vi "Prepare message set.vi"() -> (1 "Map":T3(c390), 2 "NoMessges":i32[][](array[numeric]), 3 "Array of Tx and Rx messages":T4(array[cluster]) {"ID" format="%.0x"; "DATA[0]" format="%.0x"; "DATA[1]" format="%.0x"; "DATA[2]" format="%.0x"; "DATA[3]" format="%.0x"; "DATA[4]" format="%.0x"; "DATA[5]" format="%.0x"; "DATA[6]" format="%.0x"; "DATA[7]" format="%.0x"})   [LabVIEW 2025]
uses:
  Commands.ctl
  <vilib>/Utility/file.llb/Read Delimited Spreadsheet (string).vi
panel:
  in  "Enum 3":T1=enum."MCU Reset"
  out "key not found?":bool
  out "value":T2 {"Tx und Rx"."DATA[0]" format="%.0x"; "Tx und Rx"."DATA[1]" format="%.0x"; "Tx und Rx"."DATA[2]" format="%.0x"; "Tx und Rx"."DATA[3]" format="%.0x"; "Tx und Rx"."DATA[4]" format="%.0x"; "Tx und Rx"."DATA[5]" format="%.0x"; "Tx und Rx"."DATA[6]" format="%.0x"; "Tx und Rx"."DATA[7]" format="%.0x"}
  in  "stop":bool
  out "Array":bool[](array[boolean])
  out "for debug":string[][](array[string])
  out "all rows":string[][](array[string])
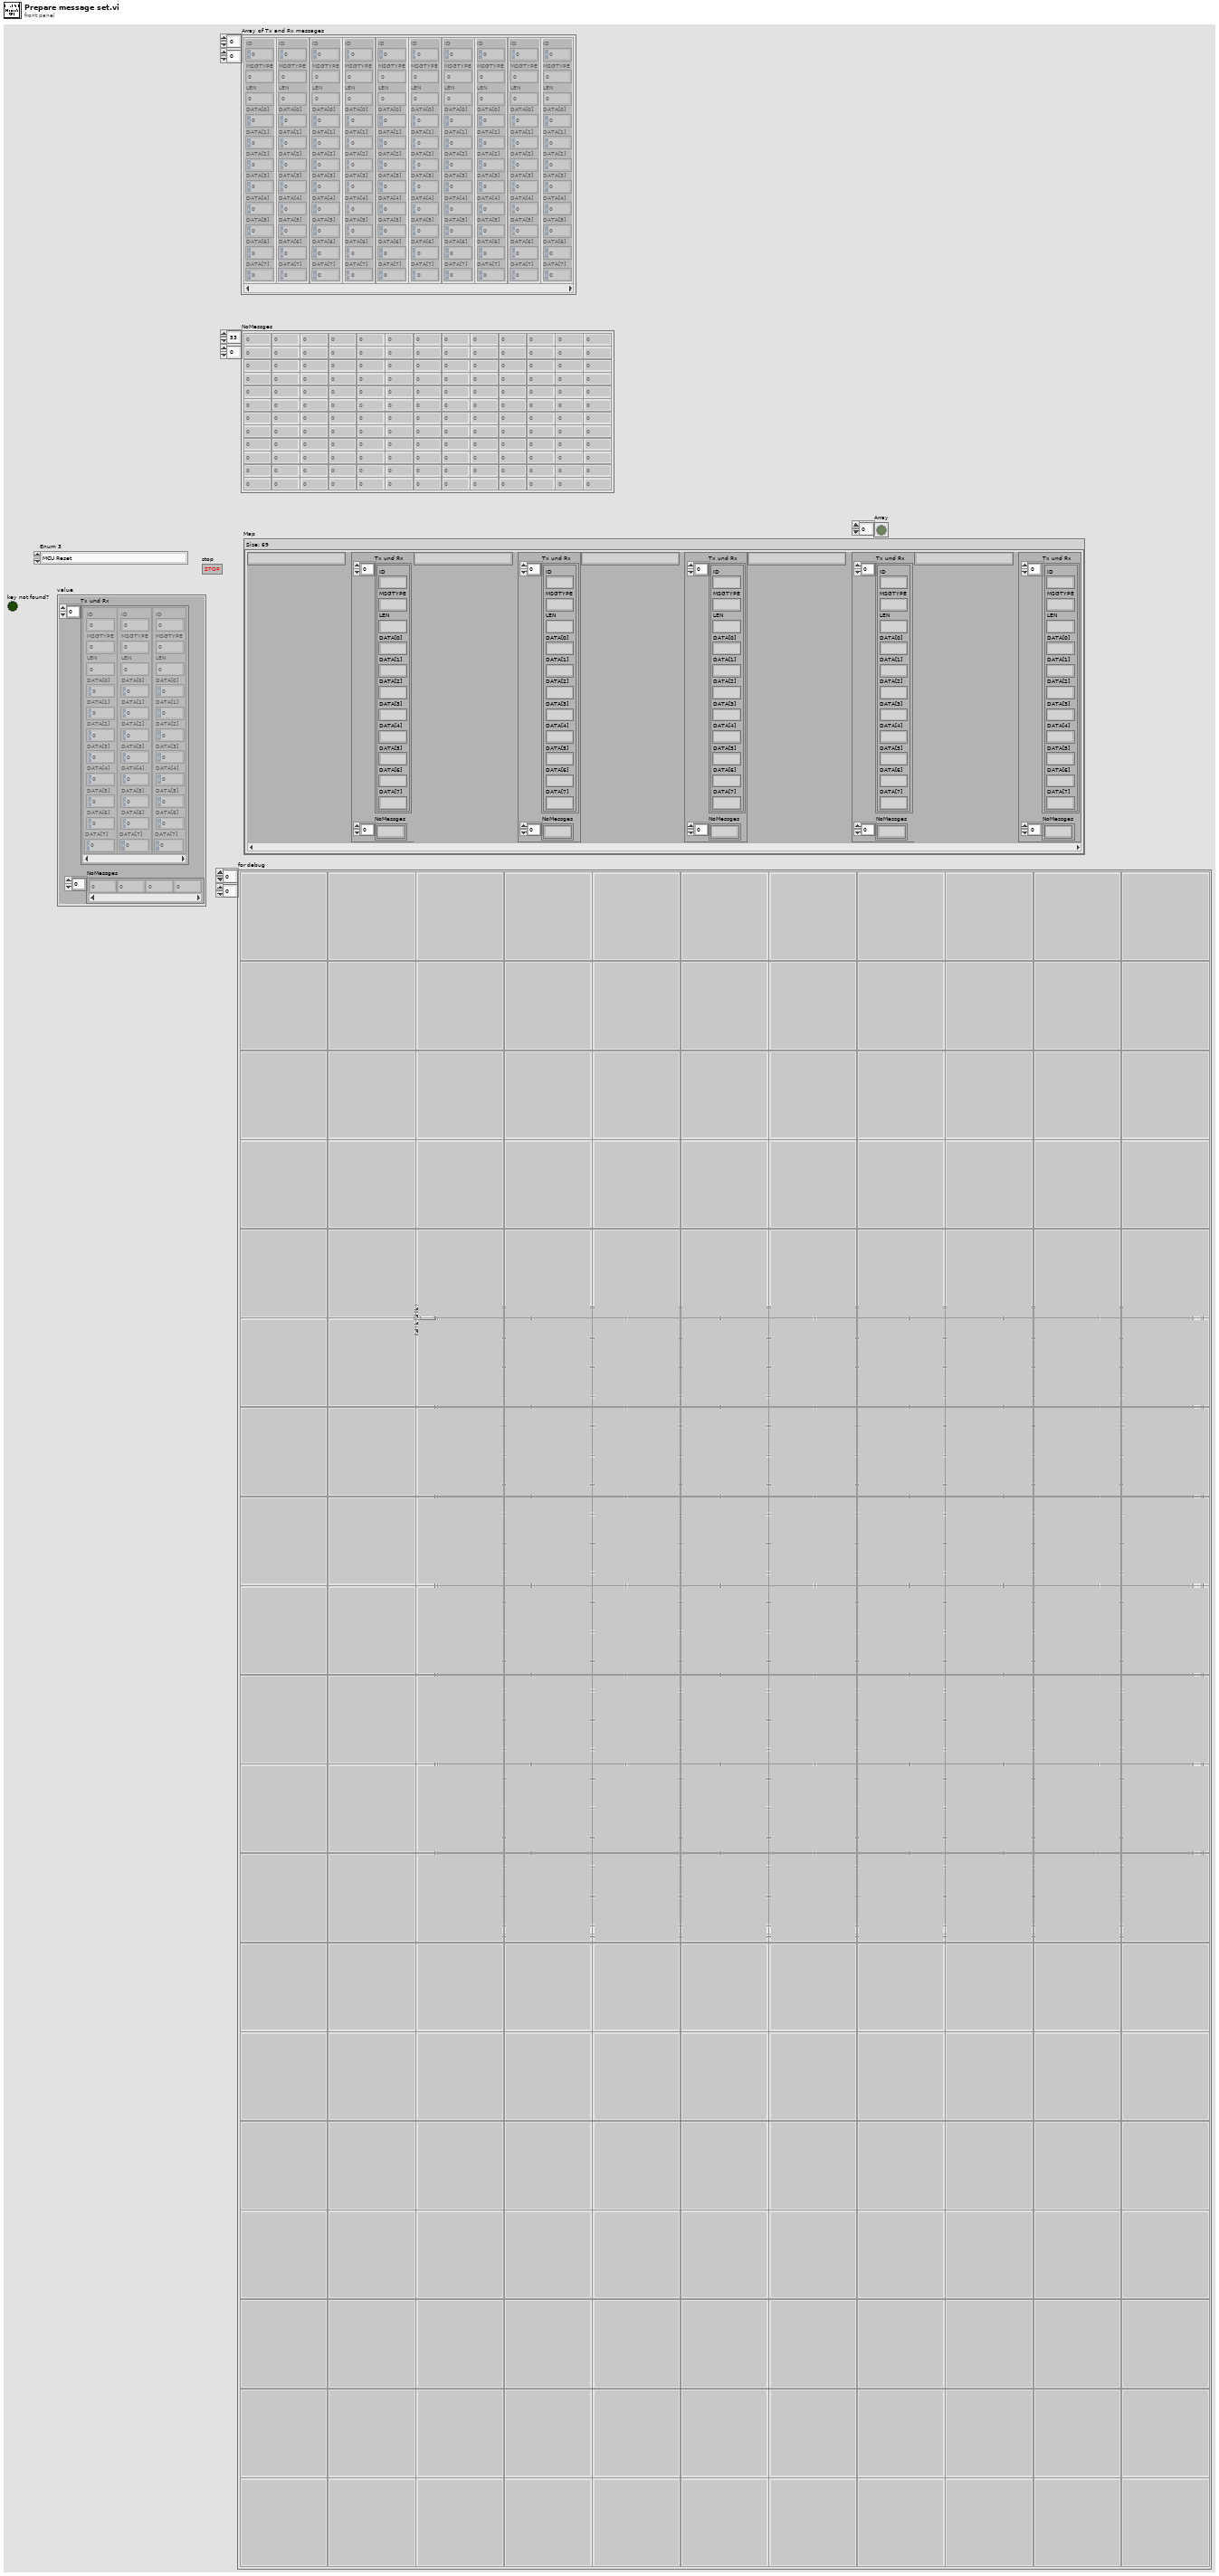
[diagram p1: front panel]
types:
  T1 = typedef "Commands.ctl" = enum16{"Nexteer connect", "Write Polarity", "Write BEMF", "Write Torque Scale Sensors T1", "Write Torque Scale Sensors T2", "Trim HW Torque Sensors T1", "Trim HW Torque Sensors T2", "Read HW Torque Trim Performed Sensors T1", "Read HW Torque Trim Performed Sensors T2", "Write EOL Offset values to defaults", "Write EOL Gain values to defaults", "Write Serial Number", "Write Hardware Part Number", "Write EPS Serial Number", "Read MEC Counter", "MCU Reset", "Read System State", "Read First Motor Position", "Manufacturing Diagnostic Defeat", "Perform Current Offset ", "Current Offset Status", "Enable Engine Run", "Perform Current Gain ", "Current Gain Status", "Disable Torque Ramp Down ", "Disable Engine Run", "Set Vehicle Speed Override", "Read Offset Values Using FD F5", "Read Gain Values Using FD F4", "Clear Nexteer NTCs", "Read Second Motor Position", "Read ECU Software ID", "Read Internal Software Version", "Read Bootloader ID", "Read Bootloader Software Version", "Read Calibration Release 0", "Read Calibration Release 1", "Read Calibration Release 2", "Read Temperature  ", "Battery Voltage  ", "Read Motor Angle 0", "Read Motor Angle 1 ", "Set Motor Torque Command ", "Read Motor Current   ", "Stop Motor Torque Command", "Read NTCs", "Read Serial Number", "Read HW Part Number", "Read Polarity", "Set NVM Access Defeat", "Read Software Release", "Read Software Build Date", "Write Single Inverter Hardware value", "Write Dual Inverter Hardware value", "Read Single Inverter HW Value", "Read Dual Inverter HW Value", "Write MEC Counter FE", "Write MEC Counter FF", "Read BEMF", "Read Torque 1 FDB6", "Read Torque 2 FDB7", "Read Torque Trim 1 FDB4", "Read Torque Trim 2 FDB5", "Write Torque Trim 1 FDB4", "Write Torque Trim 2 FDB5", "XCP connect", "Read HW Torque T1", "Read HW Torque T2", "Read Motor Speed "}
  T2 = cluster{"Tx und Rx":cluster{"ID":u32, "MSGTYPE":u8, "LEN":u8, "DATA[0]":u8, "DATA[1]":u8, "DATA[2]":u8, "DATA[3]":u8, "DATA[4]":u8, "DATA[5]":u8, "DATA[6]":u8, "DATA[7]":u8}[], "NoMessges":i32[]}
  T3 = map{string, cluster{"Tx und Rx":cluster{"ID":u32, "MSGTYPE":u8, "LEN":u8, "DATA[0]":u8, "DATA[1]":u8, "DATA[2]":u8, "DATA[3]":u8, "DATA[4]":u8, "DATA[5]":u8, "DATA[6]":u8, "DATA[7]":u8}[], "NoMessges":i32[]}}
  T4 = cluster{"ID":u32, "MSGTYPE":u8, "LEN":u8, "DATA[0]":u8, "DATA[1]":u8, "DATA[2]":u8, "DATA[3]":u8, "DATA[4]":u8, "DATA[5]":u8, "DATA[6]":u8, "DATA[7]":u8}[][]
  T5 = cluster{"ID":u32, "MSGTYPE":u8, "LEN":u8, "DATA[0]":u8, "DATA[1]":u8, "DATA[2]":u8, "DATA[3]":u8, "DATA[4]":u8, "DATA[5]":u8, "DATA[6]":u8, "DATA[7]":u8}[]
  T6 = cluster{"ID":u32, "MSGTYPE":u8, "LEN":u8, "DATA[0]":u8, "DATA[1]":u8, "DATA[2]":u8, "DATA[3]":u8, "DATA[4]":u8, "DATA[5]":u8, "DATA[6]":u8, "DATA[7]":u8}
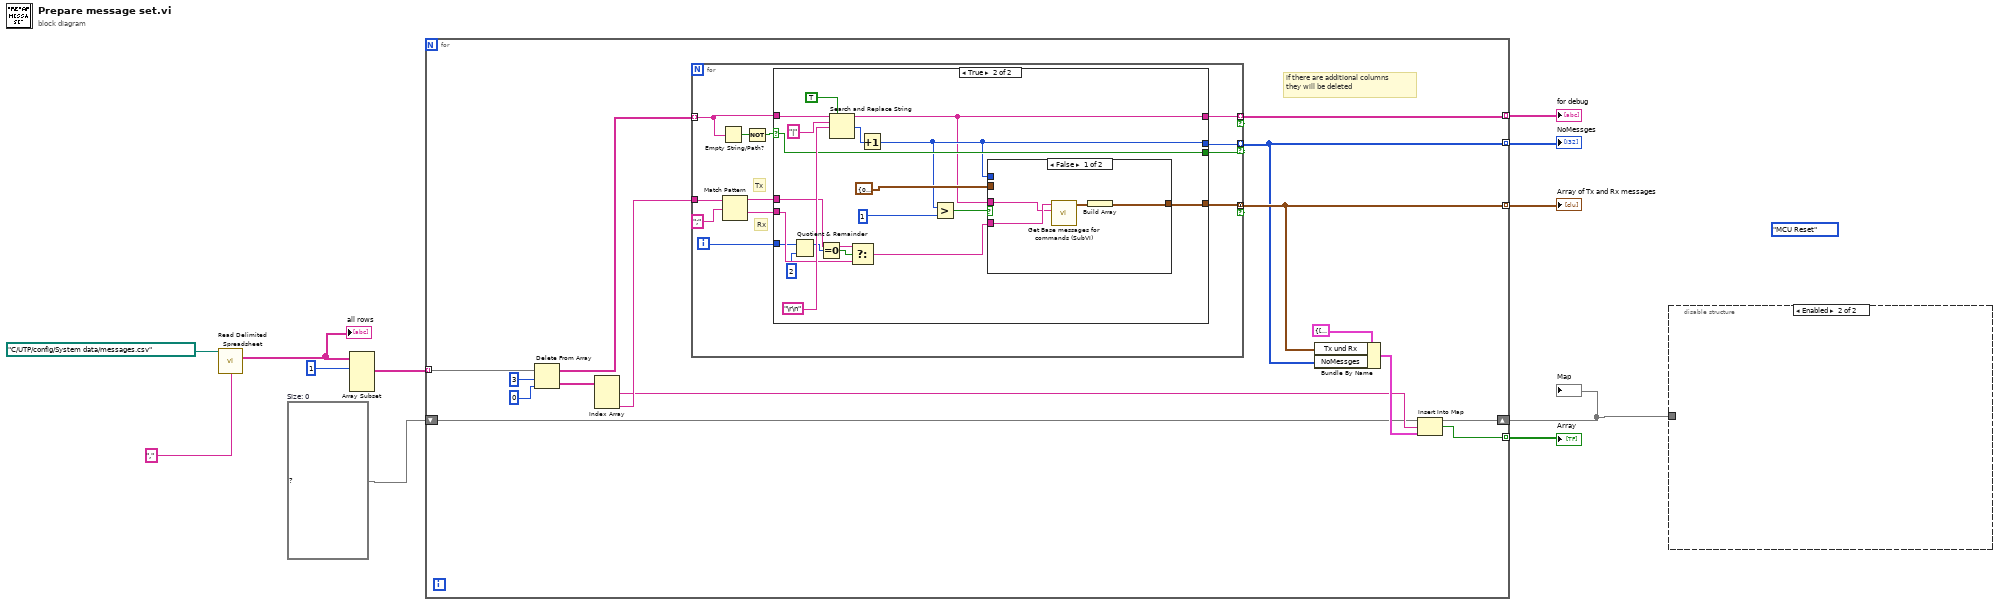
[diagram p0: block diagram]
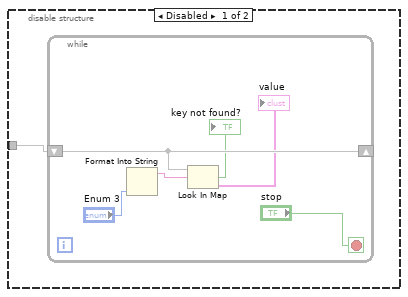
[diagram p2: hidden frame]
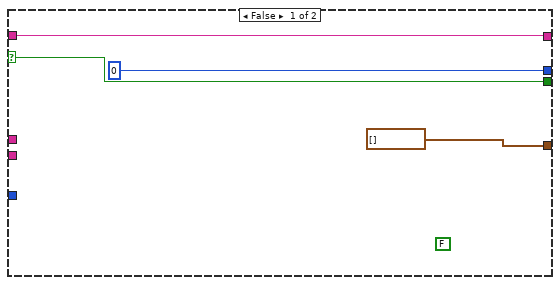
[diagram p3: hidden frame]
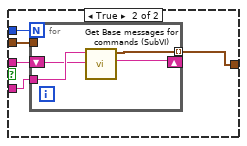
[diagram p4: hidden frame]
diagram:
  (unwired) Commands."MCU Reset" ("Enum 2")
  w3 = T3 {}  # Size: 0
  n1 = call-poly <vilib>:"Read Delimited Spreadsheet.vi"("file path (dialog if empty)"=path "C:/UTP/config/System data/messages.csv", "delimiter (\\t)"="," ("delimiter (\\t)")) -> ("all rows"=w7:string[][])  [unwired: 8 in, 5 out]
  "all rows" <- w7
  n2 = Array Subset(array=w7, index (row)=1 ("index")) -> (w5:string[][])  [unwired: 3 in]
  n3 = for {
    tunnel: w5 -> [w23] mode=indexing
    tunnel: [w26] -> w9 mode=indexing
    tunnel: [w12] -> w8 mode=indexing
    tunnel: [w14] -> w4 mode=indexing
    shift-right: [w15] -> w1
    shift-left: w3 -> [w16]
    tunnel: [w13] -> w2 mode=indexing
    # "if there are additional columns\nthey will be deleted"
    n4 = Delete From Array(array=w23, length=3, index=0) -> (deleted portion=w25:string[], array with subset deleted=w24:string[])
    n5 = Index Array(array=w25) -> (element #1=w17:string, element #3=w20:string)  [unwired: 3 in, 1 out]
    n6 = for {
      tunnel: w24 -> [w37] mode=indexing
      tunnel: [w38] -> w26 mode=indexing if=w27
      tunnel: [w34] -> w12 mode=indexing if=w27
      tunnel: w20 -> [w33]
      tunnel: [w28] -> w14 mode=concatenating if=w27
      i -> [w29]
      # "Rx"
      # "Tx"
      n7 = Empty String/Path?(string/path=w37) -> (empty?=w36:bool)
      n8 = Match Pattern(string=w33, regular expression=";") -> (before substring=w31:string, after substring=w30:string)  [unwired: 1 in, 2 out]
      n9 = Not(x=w36) -> (.not. x?=w35:bool)
      n10 = case shown="True" w35 {
        selector: w35 -> [w40 w57]
        tunnel: w37 -> [w42 w59]
        tunnel: [w42 w51] -> w38
        tunnel: [0 w54] -> w34
        tunnel: [w40 w57] -> w27
        tunnel: w31 -> [_ w50]
        tunnel: w30 -> [_ w49]
        tunnel: w29 -> [_ w48]
        tunnel: [T5 [] w44] -> w28
        frame False {
          (unwired) FALSE
        }
        frame True {
          n11 = Quotient & Remainder(x=w48, y=2) -> (x-y*floor(x/y)=w46:i32)  [unwired: 1 out]
          n12 = Equal To 0?(x=w46) -> (x = 0?=w43:bool)
          n13 = Search and Replace String(replace all?=TRUE ("replace all? (F)"), input string=w59, search string="|", replace string="\r\n") -> (result string=w51:string, number of replacements=w58:i32)  [unwired: 4 in, 2 out]
          n14 = Select(t=w50, s=w43, f=w49) -> (s? t:f=w45:string)
          n15 = Increment(x=w58) -> (x+1=w54:i32)
          n16 = Greater?(x=w54, y=1) -> (0:w52:bool)
          n17 = case shown="False" w52 {
            tunnel: T6 {"ID"=0, "MSGTYPE"=0, "LEN"=0, "DATA[0]"=0, "DATA[1]"=0, "DATA[2]"=0, "DATA[3]"=0, "DATA[4]"=0, "DATA[5]"=0, "DATA[6]"=0, "DATA[7]"=0} ("Communication") -> [_ w70]
            tunnel: w54 -> [_ w69]
            tunnel: w51 -> [w62 w68]
            tunnel: w45 -> [w63 w67]
            tunnel: [w65 w66] -> w44
            frame False {
              n18 = call "Get Base messages for commands (SubVI).vi"("result string in"=w62, "ID"=w63) -> ("Communication out"=w64:T6)  [unwired: 8 in, 1 out]
              n19 = Build Array(w64) -> (w65:T5)
            }
            frame True {
              n20 = for {
                N: w69 -> [_]
                tunnel: w70 -> [_]
                shift-right: [w74] -> _
                shift-left: w68 -> [w72]
                tunnel: w67 -> [w73]
                tunnel: [w71] -> w66 mode=indexing
                n21 = call "Get Base messages for commands (SubVI).vi"("result string in"=w72, "ID"=w73) -> ("result string out"=w74:string, "Communication out"=w71:T6)  [unwired: 8 in]
              }
            }
          }
        }
      }
    }
    n22 = Bundle By Name(cluster=T2 {"Tx und Rx"=[{"ID"=1810, "MSGTYPE"=0, "LEN"=8, "DATA[0]"=2, "DATA[1]"=16, "DATA[2]"=126, "DATA[3]"=0, "DATA[4]"=0, "DATA[5]"=0, "DATA[6]"=0, "DATA[7]"=0}, {"ID"=1808, "MSGTYPE"=0, "LEN"=8, "DATA[0]"=2, "DATA[1]"=80, "DATA[2]"=126, "DATA[3]"=0, "DATA[4]"=0, "DATA[5]"=0, "DATA[6]"=0, "DATA[7]"=0}, {"ID"=0, "MSGTYPE"=0, "LEN"=0, "DATA[0]"=0, "DATA[1]"=0, "DATA[2]"=0, "DATA[3]"=0, "DATA[4]"=0, "DATA[5]"=0, "DATA[6]"=0, "DATA[7]"=0}, {"ID"=0, "MSGTYPE"=0, "LEN"=0, "DATA[0]"=0, "DATA[1]"=0, "DATA[2]"=0, "DATA[3]"=0, "DATA[4]"=0, "DATA[5]"=0, "DATA[6]"=0, "DATA[7]"=0}, {"ID"=0, "MSGTYPE"=0, "LEN"=0, "DATA[0]"=0, "DATA[1]"=0, "DATA[2]"=0, "DATA[3]"=0, "DATA[4]"=0, "DATA[5]"=0, "DATA[6]"=0, "DATA[7]"=0}, {"ID"=0, "MSGTYPE"=0, "LEN"=0, "DATA[0]"=0, "DATA[1]"=0, "DATA[2]"=0, "DATA[3]"=0, "DATA[4]"=0, "DATA[5]"=0, "DATA[6]"=0, "DATA[7]"=0}, {"ID"=0, "MSGTYPE"=0, "LEN"=0, "DATA[0]"=0, "DATA[1]"=0, "DATA[2]"=0, "DATA[3]"=0, "DATA[4]"=0, "DATA[5]"=0, "DATA[6]"=0, "DATA[7]"=0}, {"ID"=0, "MSGTYPE"=0, "LEN"=0, "DATA[0]"=0, "DATA[1]"=0, "DATA[2]"=0, "DATA[3]"=0, "DATA[4]"=0, "DATA[5]"=0, "DATA[6]"=0, "DATA[7]"=0}, {"ID"=0, "MSGTYPE"=0, "LEN"=0, "DATA[0]"=0, "DATA[1]"=0, "DATA[2]"=0, "DATA[3]"=0, "DATA[4]"=0, "DATA[5]"=0, "DATA[6]"=0, "DATA[7]"=0}, {"ID"=0, "MSGTYPE"=0, "LEN"=0, "DATA[0]"=0, "DATA[1]"=0, "DATA[2]"=0, "DATA[3]"=0, "DATA[4]"=0, "DATA[5]"=0, "DATA[6]"=0, "DATA[7]"=0}, {"ID"=0, "MSGTYPE"=0, "LEN"=0, "DATA[0]"=0, "DATA[1]"=0, "DATA[2]"=0, "DATA[3]"=0, "DATA[4]"=0, "DATA[5]"=0, "DATA[6]"=0, "DATA[7]"=0}, {"ID"=0, "MSGTYPE"=0, "LEN"=0, "DATA[0]"=0, "DATA[1]"=0, "DATA[2]"=0, "DATA[3]"=0, "DATA[4]"=0, "DATA[5]"=0, "DATA[6]"=0, "DATA[7]"=0}, {"ID"=0, "MSGTYPE"=0, "LEN"=0, "DATA[0]"=0, "DATA[1]"=0, "DATA[2]"=0, "DATA[3]"=0, "DATA[4]"=0, "DATA[5]"=0, "DATA[6]"=0, "DATA[7]"=0}, {"ID"=0, "MSGTYPE"=0, "LEN"=0, "DATA[0]"=0, "DATA[1]"=0, "DATA[2]"=0, "DATA[3]"=0, "DATA[4]"=0, "DATA[5]"=0, "DATA[6]"=0, "DATA[7]"=0}, {"ID"=0, "MSGTYPE"=0, "LEN"=0, "DATA[0]"=0, "DATA[1]"=0, "DATA[2]"=0, "DATA[3]"=0, "DATA[4]"=0, "DATA[5]"=0, "DATA[6]"=0, "DATA[7]"=0}, {"ID"=0, "MSGTYPE"=0, "LEN"=0, "DATA[0]"=0, "DATA[1]"=0, "DATA[2]"=0, "DATA[3]"=0, "DATA[4]"=0, "DATA[5]"=0, "DATA[6]"=0, "DATA[7]"=0}, {"ID"=0, "MSGTYPE"=0, "LEN"=0, "DATA[0]"=0, "DATA[1]"=0, "DATA[2]"=0, "DATA[3]"=0, "DATA[4]"=0, "DATA[5]"=0, "DATA[6]"=0, "DATA[7]"=0}], "NoMessges"=[1, 1, 0, 0, 0, 0]}, "Tx und Rx"=w14, "NoMessges"=w12) -> (w19:T2)
    n23 = Insert Into Map(map in=w16, key=w17, value=w19) -> (map out=w15:T3, key already included?=w13:bool)  [unwired: 1 out]
  }
  "for debug" <- w9
  "NoMessges" <- w8
  "Array of Tx and Rx messages" <- w4
  "Map" <- w1
  "Array" <- w2
  n24 = disable-structure shown="Enabled" {
    disable-tunnel: w1 -> [w75 _]
    frame Disabled {
      n25 = while {
        shift-right: [w80] -> _
        shift-left: w75 -> [w80]
        stop <- "stop" stop-if-true
        n26 = Format Into String("Enum 3") -> (resulting string=w78:string)  [unwired: 3 in, 1 out]
        n27 = Look In Map(map=w80, key=w78) -> (key not found?=→"key not found?":bool, value=→"value":T2)  [unwired: 1 in]
      }
    }
    frame Enabled {
    }
  }
